vi "Get App Port.vi"(8 "error in (no error)":errorcluster, 11 "App Ref":refnum<vi>) -> (0 "error out":errorcluster, 2 "Port":string, 3 "App Ref out":refnum<vi>)   [LabVIEW 2020, in "MacroAssert.lvlib"]
doc: "Outputs the port of <B>App Ref</B>."
uses:
  MacroAssert.lvlib
  <vilib>/Utility/config.llb/NI_LVConfig.lvlib
  <vilib>/Utility/config.llb/Read Key (I32).vi
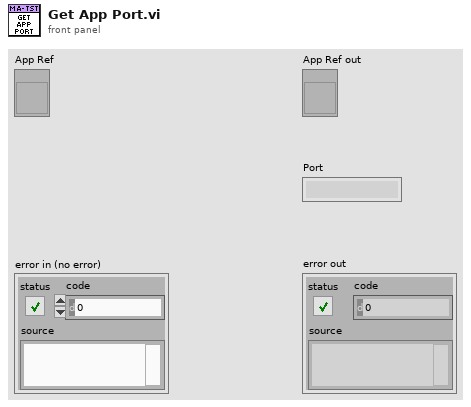
[diagram p1: front panel]
types:
  T1 = enum32{"invalid app kind", "Development System", "Run Time System", "Student Edition", "Embedded LabVIEW", "Evaluation", "Custom"}
  T2 = typedef "NI_LVConfig.lvlib/Config Data RefNum.ctl" = refnum<k1>
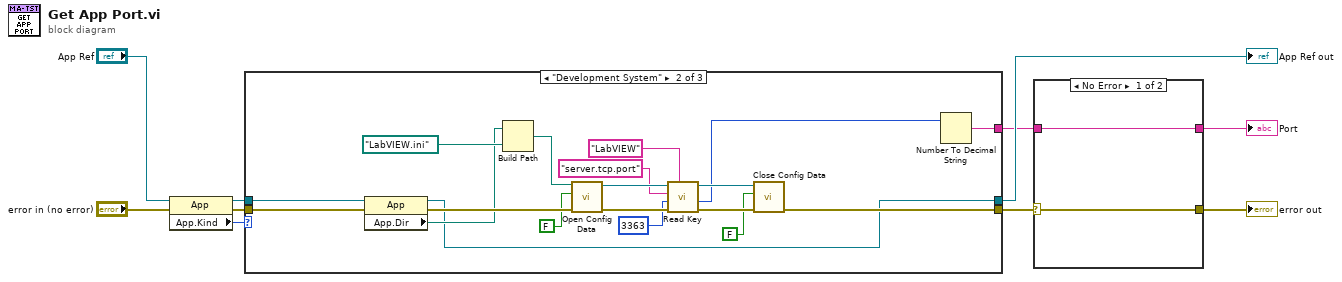
[diagram p0: block diagram]
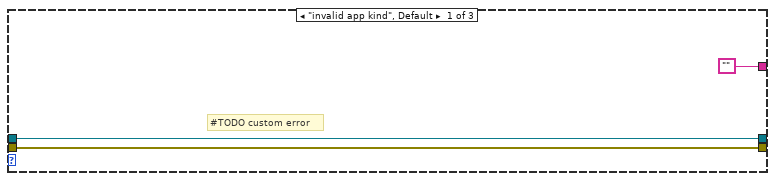
[diagram p3: hidden frame]
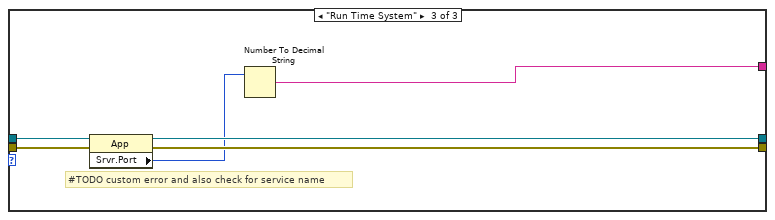
[diagram p4: hidden frame]
diagram:
  n1 = property class="App"(reference="App Ref", error in="error in (no error)") -> (reference out=w5:refnum<vi>, error out=w10:errorcluster, "App.Kind"=w3:T1)
  n2 = case shown="\"Development System\"" w3 {
    tunnel: w10 -> [w13 w30 w38]
    tunnel: w5 -> [w12 w27 w36]
    tunnel: [w13 w28 w37] -> w7
    tunnel: ["" w24 w33] -> w2
    tunnel: [w12 w14 w35] -> w4
    frame "invalid app kind", Default {
      # "#TODO custom error"
    }
    frame "Development System" {
      n3 = property class="App"(reference=w27, error in=w30) -> (reference out=w14:refnum<vi>, error out=w29:errorcluster, "App.Dir"=w18:path)
      n4 = Build Path(base path=w18, name or relative path=path "LabVIEW.ini") -> (appended path=w23:path)
      n5 = call <vilib>:"Open Config Data.vi"("error in (no error)"=w29, "create file if necessary (T)"=FALSE, "configuration file path"=w23) -> ("error out"=w31:errorcluster, "refnum"=w26:T2)  [unwired: 6 in, 1 out]
      n6 = call-poly <vilib>:"Read Key.vi"("section"="LabVIEW", "error in (no error)"=w31, "default value"=3363, "key"="server.tcp.port", "refnum"=w26) -> ("error out"=w32:errorcluster, "value"=w15:i32, "refnum out"=w25:T2)  [unwired: 3 in, 1 out]
      n7 = call <vilib>:"Close Config Data.vi"("error in (no error)"=w32, "write file if changed (T)"=FALSE, "refnum"=w25) -> ("error out"=w28:errorcluster)  [unwired: 7 in, 1 out]
      n8 = Number To Decimal String(number=w15) -> (decimal integer string=w24:string)  [unwired: 1 in]
    }
    frame "Run Time System" {
      # "#TODO custom error and also check for service name"
      n9 = property class="App"(reference=w36, error in=w38) -> (reference out=w35:refnum<vi>, error out=w37:errorcluster, "Srvr.Port"=w34:u32)
      n10 = Number To Decimal String(number=w34) -> (decimal integer string=w33:string)  [unwired: 1 in]
    }
  }
  "App Ref out" <- w4
  n11 = case shown="No Error" w7 {
    selector: w7 -> [w40 w41]
    tunnel: [w40 w41] -> w8
    tunnel: w2 -> [w39 _]
    tunnel: [w39 _] -> w1
    frame No Error {
    }
    frame Error {
    }
  }
  "error out" <- w8
  "Port" <- w1
